vi "main_engine.vi"() -> ()   [LabVIEW 2023]
uses:
  <vilib>/numeric/Random Number (Range) U64.vi
  <vilib>/numeric/sub_Random U32.vi
  <vilib>/sound2/lvsound2.llb/Sound Output Set Volume (Single).vi
panel:
  out "Score":i32
  out "Combo":i32
  out "Multiplier":i32=1
  in  "Buttons":bool[](array[boolean])=[FALSE, FALSE, FALSE, TRUE, FALSE, FALSE, FALSE, FALSE, FALSE, FALSE, FALSE, FALSE, FALSE, FALSE, FALSE, FALSE]
  in  "stop (F)":bool
  in  "Mode":enum16{"Simulated", "Hardware"}(ring)
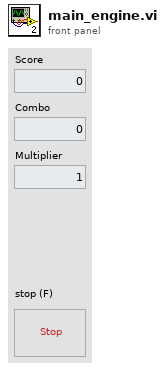
[diagram p1: front panel]
types:
  T1 = typedef "Sound Output Task ID.ctl" = u32
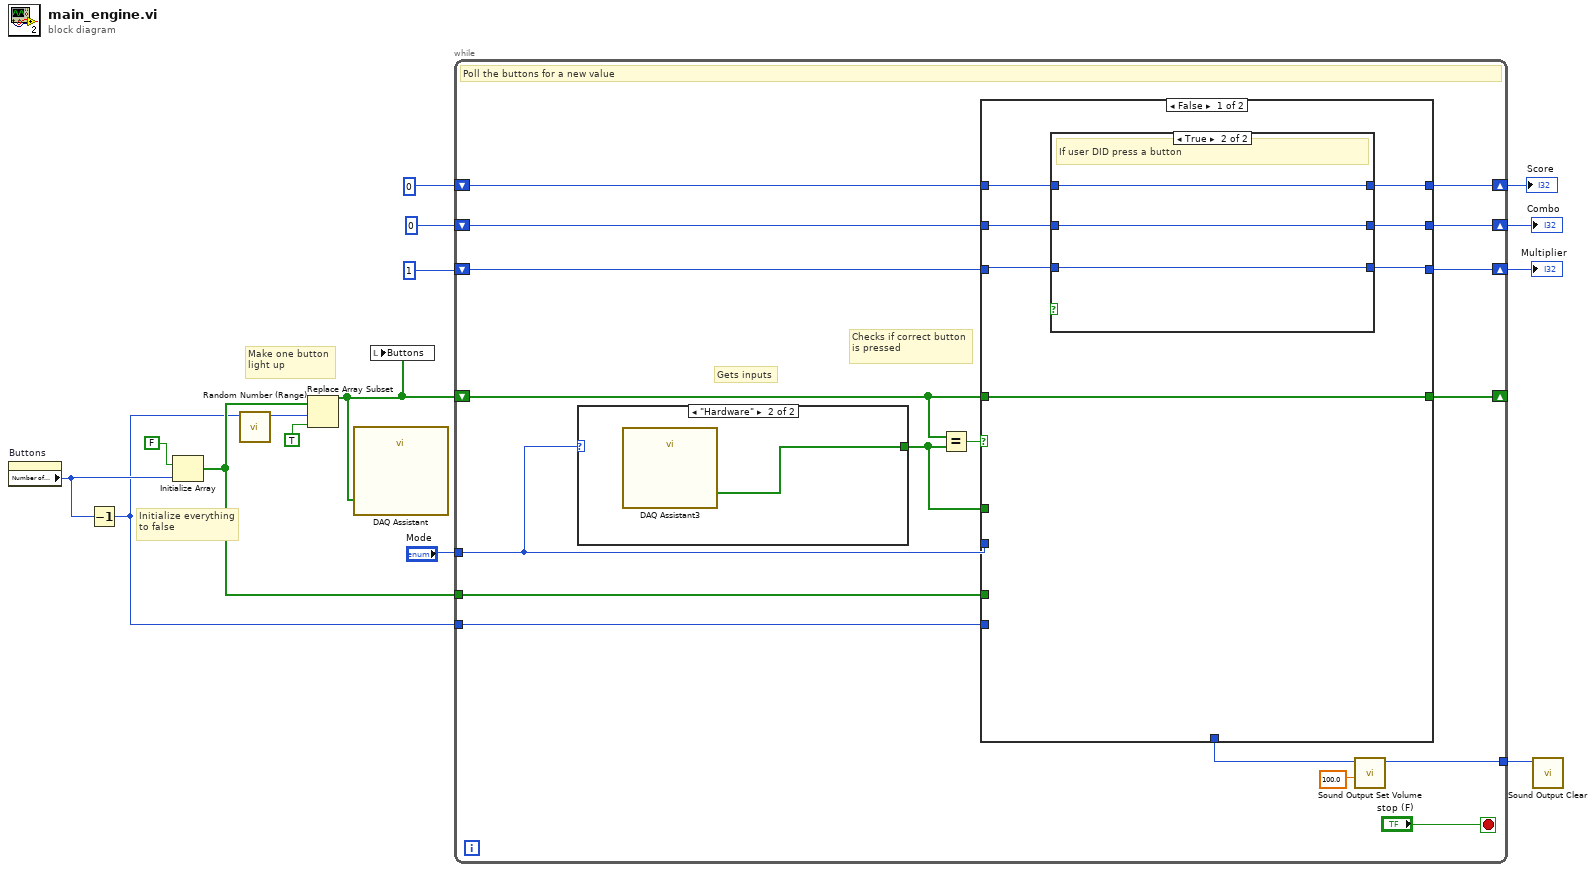
[diagram p0: block diagram]
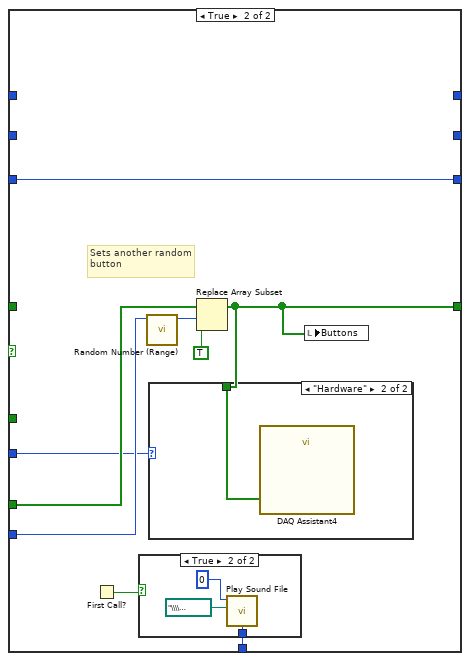
[diagram p3: hidden frame]
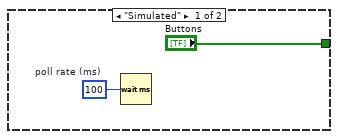
[diagram p6: hidden frame]
diagram:
  # "Initialize everything to false"
  # "Make one button light up"
  n1 = property on="Buttons" class="Arr (strict)"() -> ("Number of Columns"=w9:u32)  [unwired: 2 in, 2 out]
  n2 = Decrement(x=w9) -> (x-1=w8:u32)
  n3 = Initialize Array(FALSE, w9) -> (w12:bool[])
  n4 = call-poly <vilib>:"Random Number (Range).vi"("upper bound (100)"=w8) -> ("number"=w14:u64)  [unwired: 10 in]
  n5 = Replace Array Subset(array=w12, new element=TRUE ("new element/subarray"), index=w14) -> (w10:bool[])
  n6 = call "DAQ Assistant"("data"=w10) -> ()  [unwired: 17 in, 2 out]
  n7 = local write "Buttons"(w10) -> ()
  n8 = while {
    tunnel: w12 -> [w29]
    shift-right: [w30] -> _
    shift-left: w10 -> [w31]
    tunnel: w8 -> [w28]
    tunnel: "Mode" -> [w26]
    tunnel: [w24] -> w7
    shift-right: [w20] -> w5
    shift-left: 1 -> [w21]
    shift-right: [w19] -> w4
    shift-left: 0 -> [w18]
    shift-right: [w17] -> w2
    shift-left: 0 -> [w16]
    stop <- "stop (F)" stop-if-true
    # "Checks if correct button is pressed"
    # "Gets inputs"
    # "Poll the buttons for a new value"
    n9 = case shown="\"Hardware\"" w26 {
      tunnel: ["Buttons" w58] -> w27
      frame "Simulated" {
        w57 = u32 100  # poll rate (ms)
        n10 = Wait (ms)(milliseconds to wait=w57) -> ()  [unwired: 1 out]
      }
      frame "Hardware" {
        n11 = call "DAQ Assistant3"() -> ("data"=w58:bool[])  [unwired: 17 in, 2 out]
      }
    }
    n12 = Equal?(x=w31, y=w27) -> (x = y?=w32:bool)
    n13 = case shown="False" w32 {
      tunnel: w31 -> [w39 _]
      tunnel: [w39 w50] -> w30
      tunnel: w29 -> [_ w49]
      tunnel: w27 -> [_ _]
      tunnel: w28 -> [_ w51]
      tunnel: w26 -> [_ w48]
      tunnel: [_ w45] -> w22
      tunnel: w21 -> [w33 w43]
      tunnel: [w34 w43] -> w20
      tunnel: [w35 _] -> w19
      tunnel: w18 -> [w36 _]
      tunnel: [w38 _] -> w17
      tunnel: w16 -> [w37 _]
      frame False {
        # "Button value did not change"
        n14 = case shown="True" {
          selector: _ -> [_ _]
          tunnel: [_ w42] -> w38
          tunnel: w37 -> [_ w42]
          tunnel: [_ w41] -> w35
          tunnel: w36 -> [_ w41]
          tunnel: [_ w40] -> w34
          tunnel: w33 -> [_ w40]
          frame False {
          }
          frame True {
            # "If user DID press a button"
          }
        }
      }
      frame True {
        # "Sets another random button"
        # "Button value changed, see if they clicked the correct button."
        n15 = First Call?() -> (First Call?: T/F=w44:bool)
        n16 = case shown="True" w44 {
          tunnel: [_ w52] -> w45
          frame False {
          }
          frame True {
            n17 = call <vilib>:"Play Sound File.vi"("path"=path "\\\\bingus-dev\\P/misc/sarah-hardware-fun/hackathon-stuff/dependencies/eye-of-the-tiger-8bit.wav", "device ID"=u32 0) -> ("task ID"=w52:T1)  [unwired: 8 in, 1 out]
          }
        }
        n18 = call-poly <vilib>:"Random Number (Range).vi"("upper bound (100)"=w51) -> ("number"=w46:u64)  [unwired: 10 in]
        n19 = Replace Array Subset(array=w49, new element=TRUE ("new element/subarray"), index=w46) -> (w50:bool[])
        n20 = case shown="\"Hardware\"" w48 {
          tunnel: w50 -> [_ w55]
          frame "Simulated" {
          }
          frame "Hardware" {
            n21 = call "DAQ Assistant4"("data"=w55) -> ()  [unwired: 17 in, 2 out]
          }
        }
        n22 = local write "Buttons"(w50) -> ()
      }
    }
    n23 = call-poly <vilib>:"Sound Output Set Volume.vi"("volume"=100.0 ("Slide"), "task ID"=w22) -> ("task ID out"=w24:T1)  [unwired: 8 in, 1 out]
  }
  "Multiplier" <- w5
  "Combo" <- w4
  "Score" <- w2
  n24 = call <vilib>:"Sound Output Clear.vi"("task ID"=w7) -> ()  [unwired: 10 in, 1 out]
